vi "Balance Update.vi"(8 "error in (no error)":errorcluster, 11 "Bal.Update":T1=enum."FastCash") -> (0 "error out":errorcluster)   [LabVIEW 2013, in "ConfigDBLib.lvlib"]
uses:
  ConfigDBLib.lvlib
  Private Controls/Balance Update.ctl
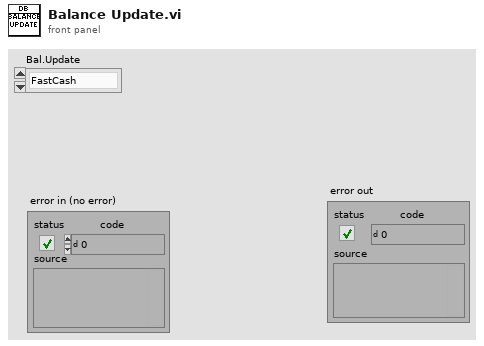
[diagram p1: front panel]
types:
  T1 = typedef "ConfigDBLib.lvlib/Balance Update.ctl" = enum16{"Balance", "Deposit", "Withdrawal", "FastCash"}
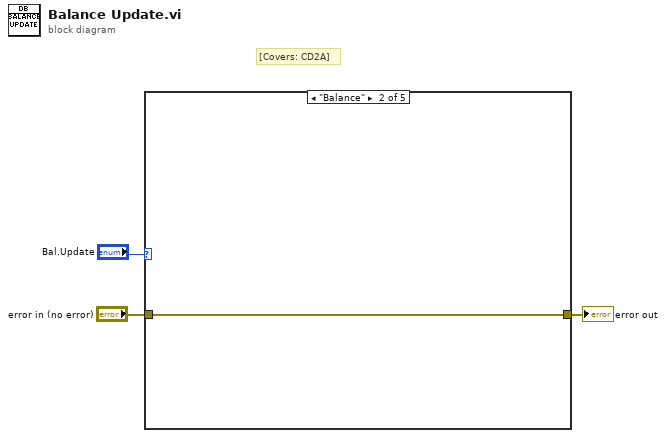
[diagram p0: block diagram]
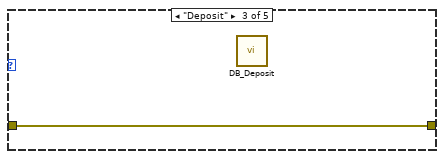
[diagram p3: hidden frame]
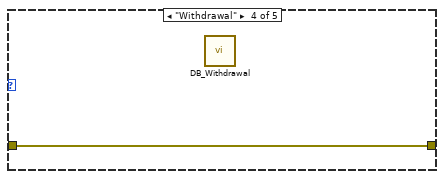
[diagram p4: hidden frame]
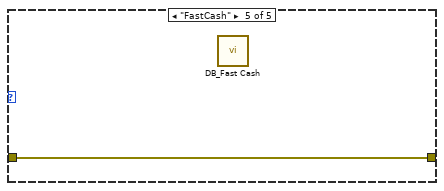
[diagram p5: hidden frame]
diagram:
  # "[Covers: CD2A]"
  n1 = case shown="\"Balance\"" "Bal.Update" {
    tunnel: [w4 w5 w6 w7 w8] -> w1
    tunnel: "error in (no error)" -> [w4 w5 w6 w7 w8]
    frame Default {
    }
    frame "Balance" {
    }
    frame "Deposit" {
      n2 = call "DB_Deposit.vi"() -> ()  [unwired: 12 in]
    }
    frame "Withdrawal" {
      n3 = call "DB_Withdrawal.vi"() -> ()  [unwired: 12 in]
    }
    frame "FastCash" {
      n4 = call "DB_Fast Cash.vi"() -> ()  [unwired: 12 in]
    }
  }
  "error out" <- w1
